vi "BRig_RT__Case_Exp__State_initTrial__LC_Select__v18.vi"(6 "input_arrTrig":bool[](array[boolean]), 8 "input_dataTrial":u16[][](array[numeric]), 9 "input_dataExp":u16[](array[numeric]), 10 "input_dataLC":u16[](array[numeric]), 11 "input_dataCurrent":u16[](array[numeric])) -> (0 "output_dataTrial":u16[][](array[numeric]), 3 "output_dataCurrent":u16[](array[numeric]), 4 "output_arrTrig":bool[](array[boolean]))   [LabVIEW 2014]
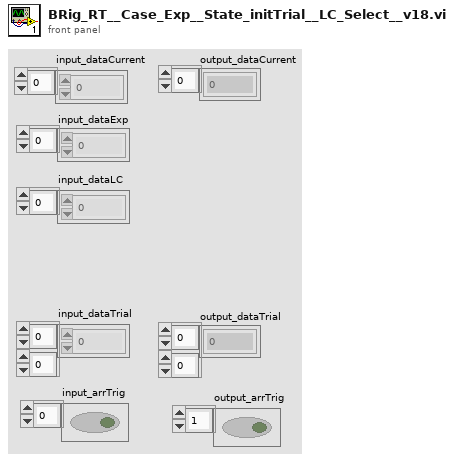
[diagram p1: front panel]
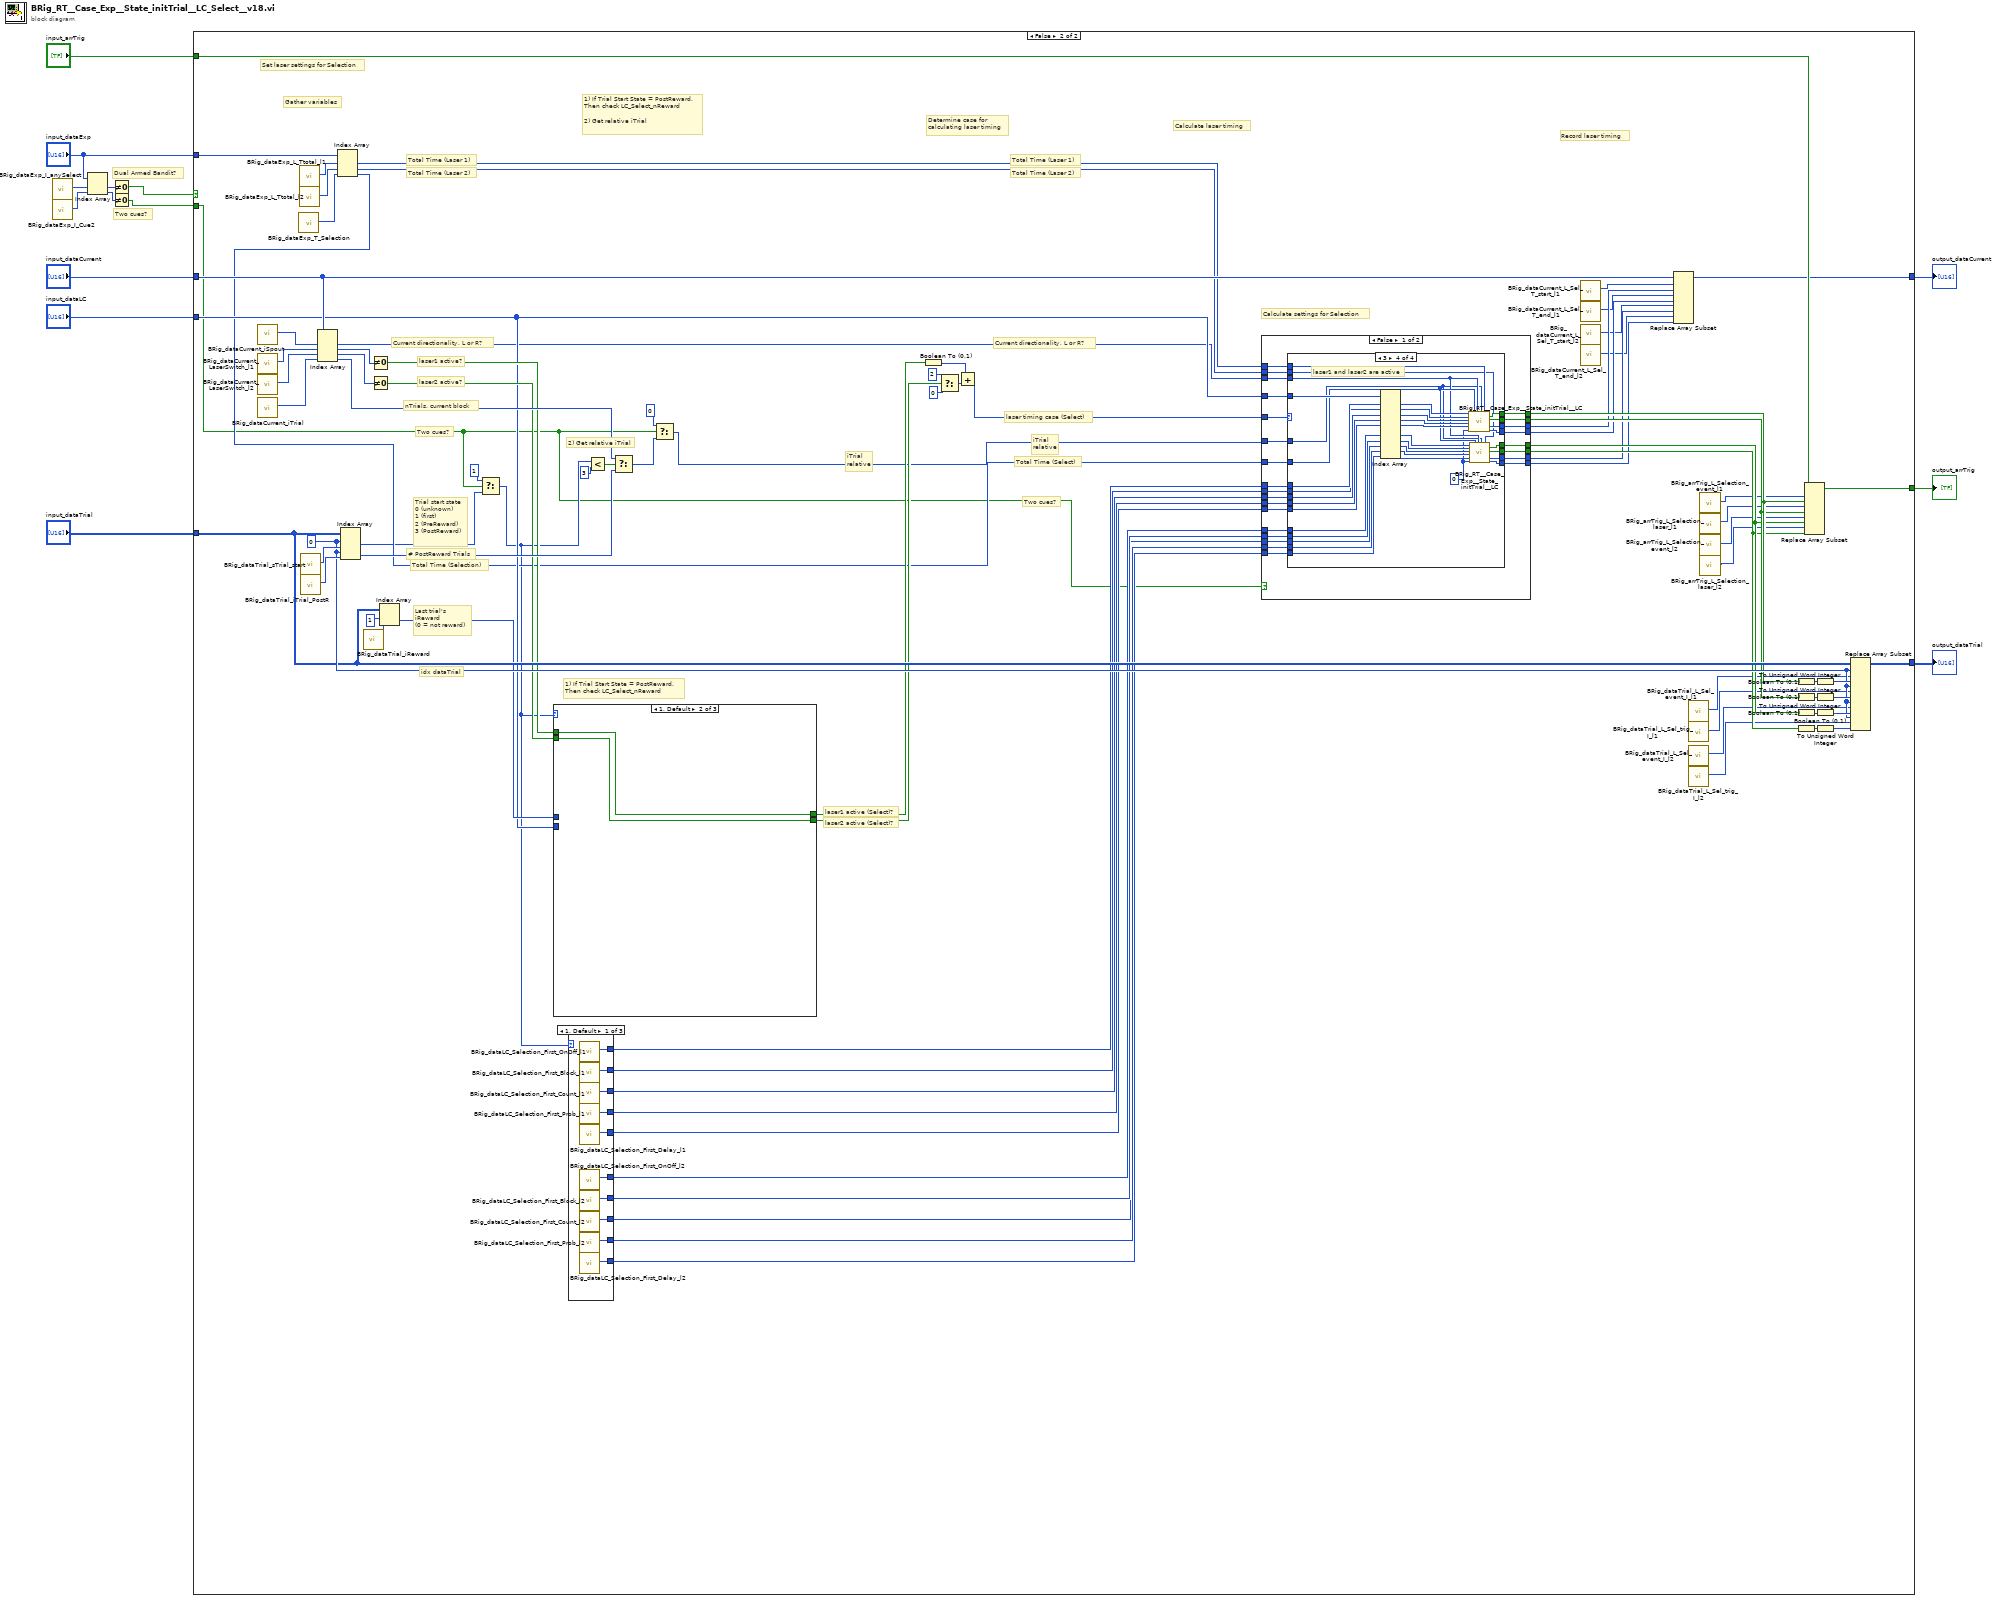
[diagram p0: block diagram]
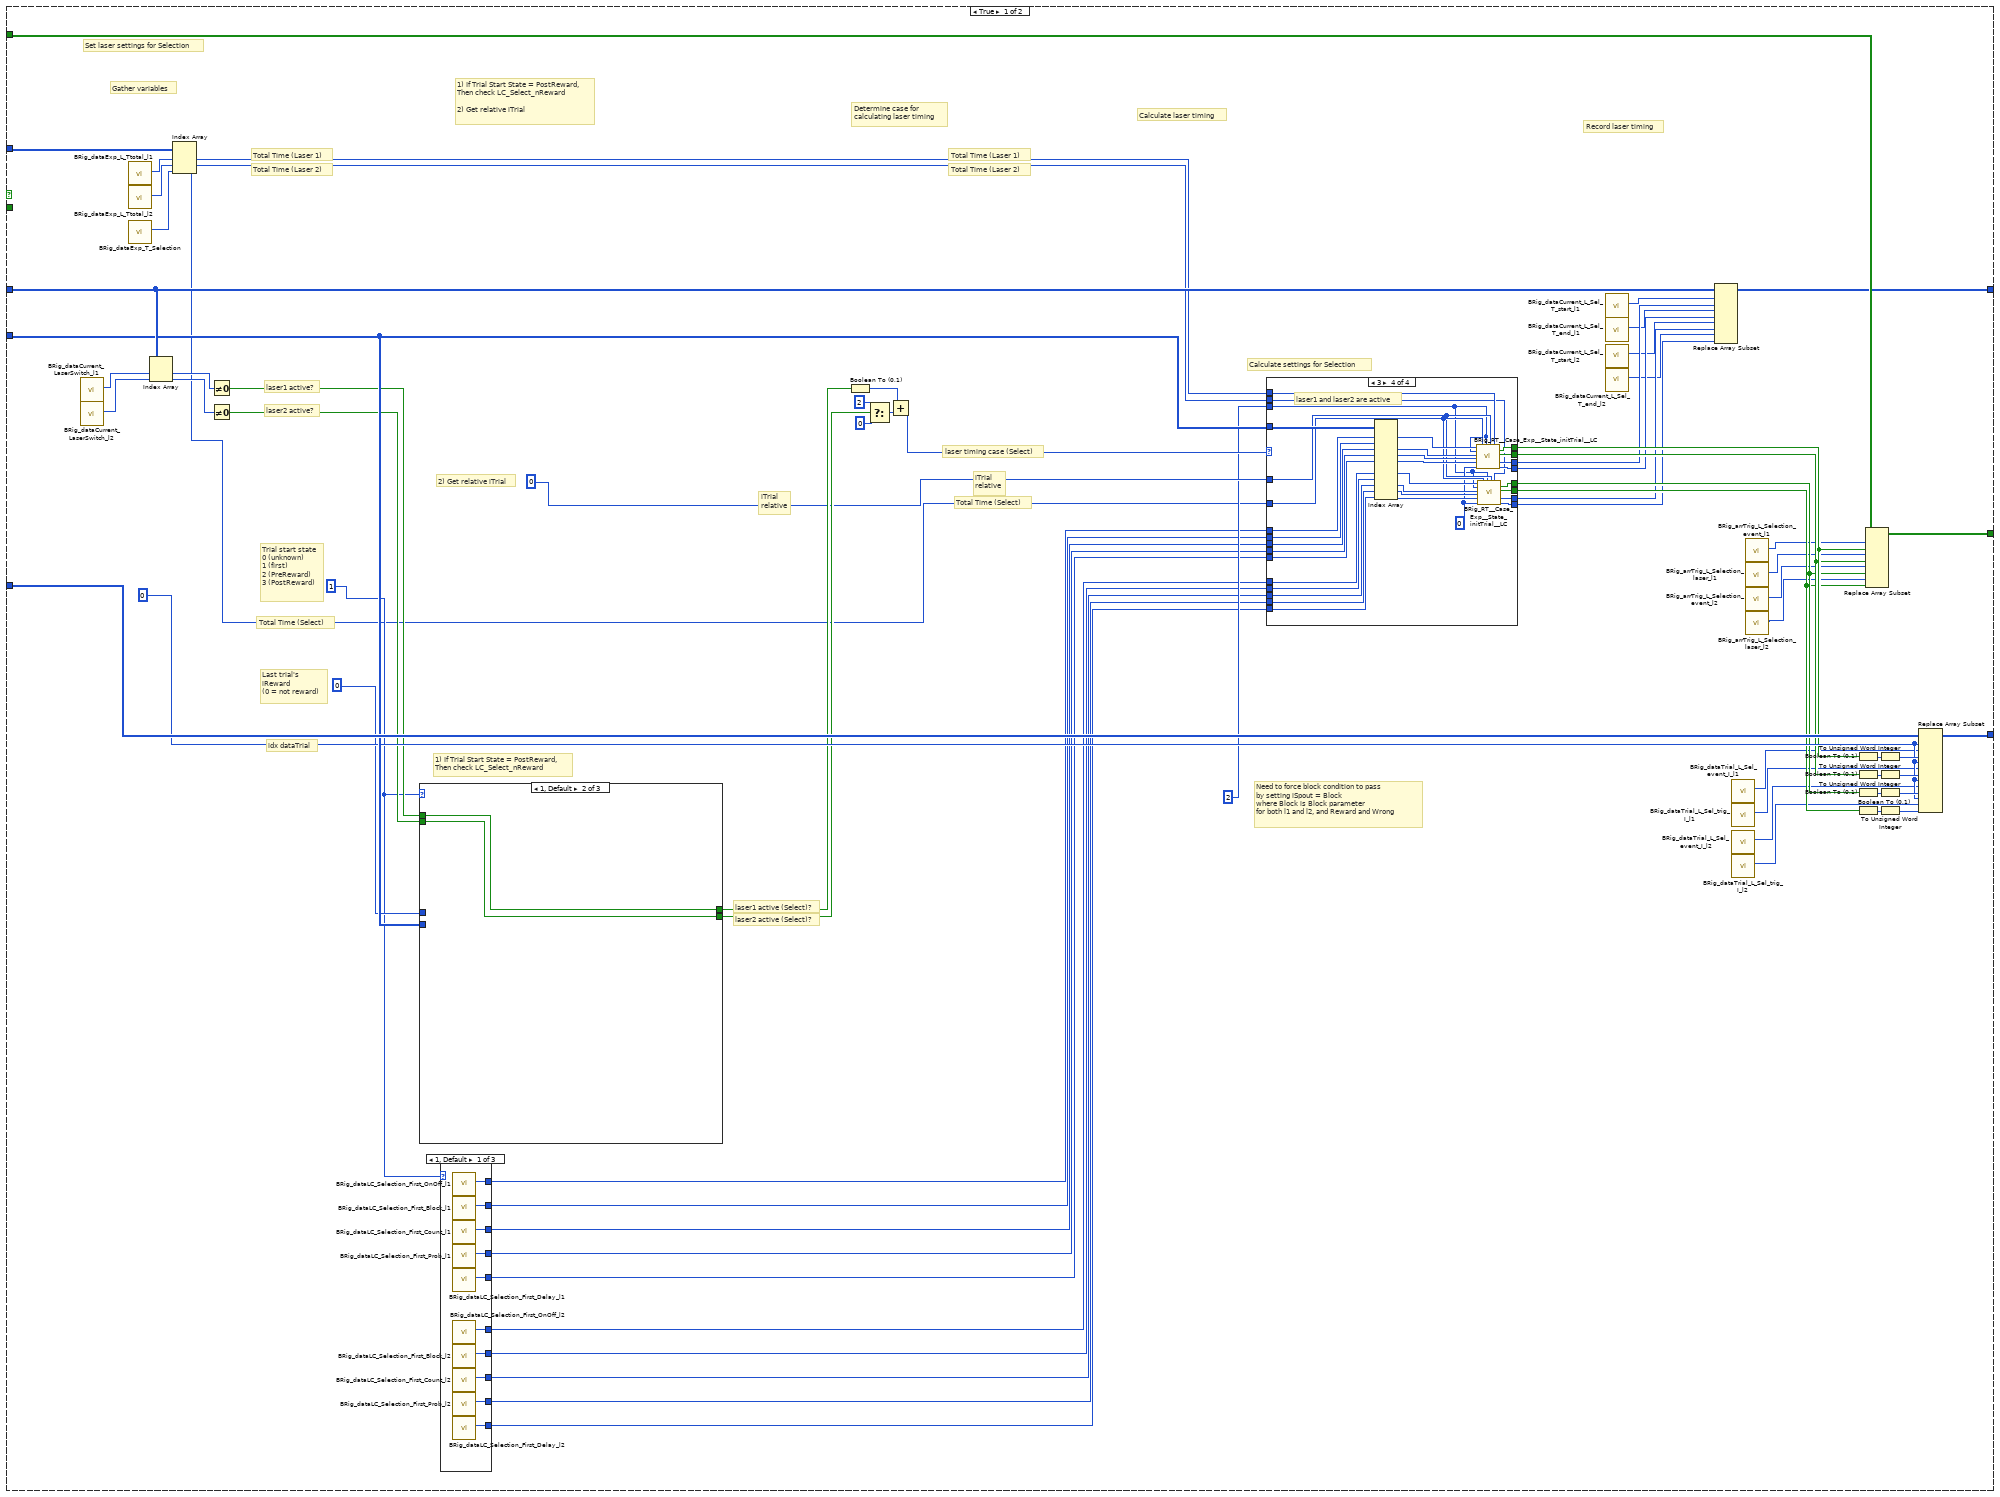
[diagram p2: hidden frame]
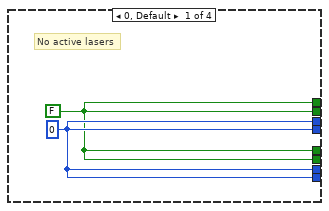
[diagram p3: hidden frame]
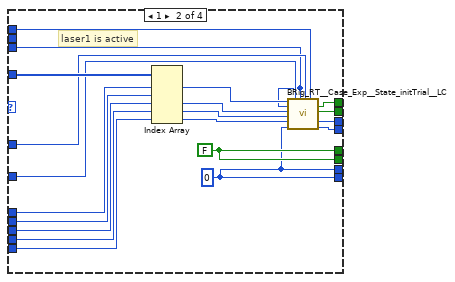
[diagram p4: hidden frame]
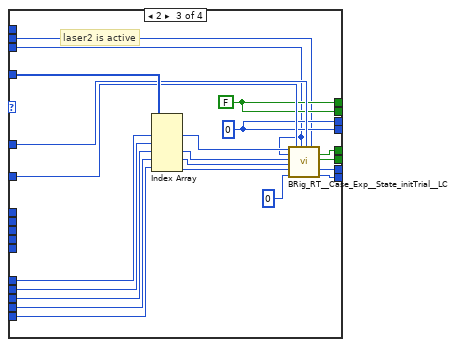
[diagram p5: hidden frame]
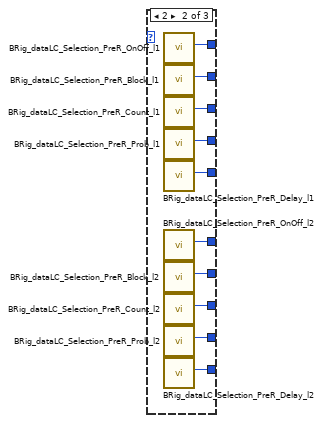
[diagram p6: hidden frame]
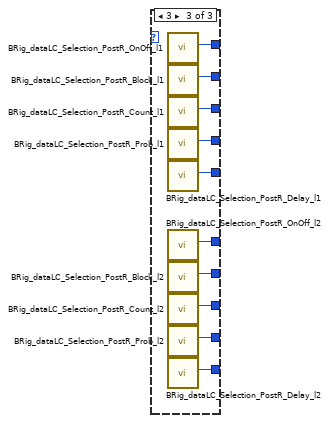
[diagram p7: hidden frame]
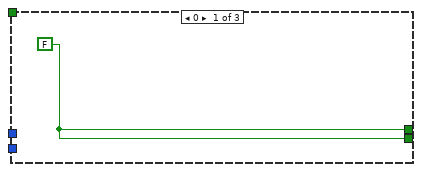
[diagram p8: hidden frame]
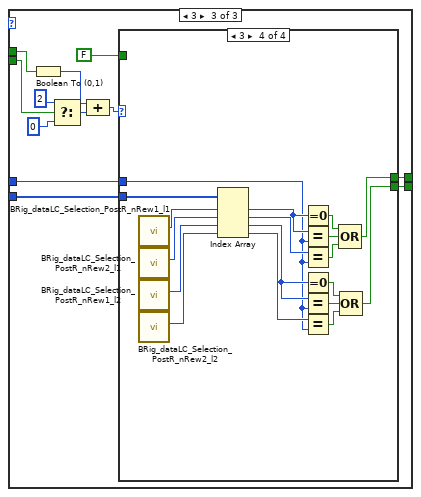
[diagram p9: hidden frame]
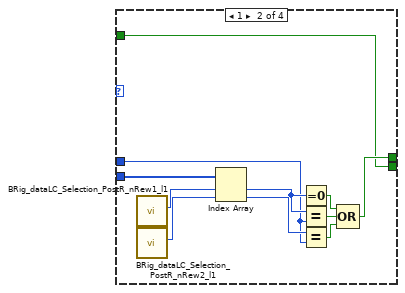
[diagram p11: hidden frame]
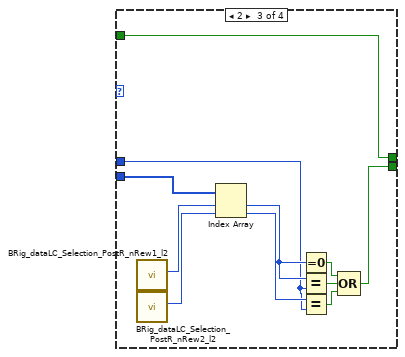
[diagram p12: hidden frame]
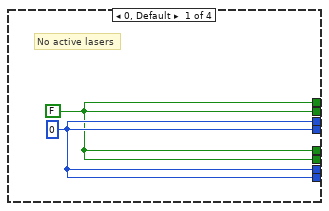
[diagram p13: hidden frame]
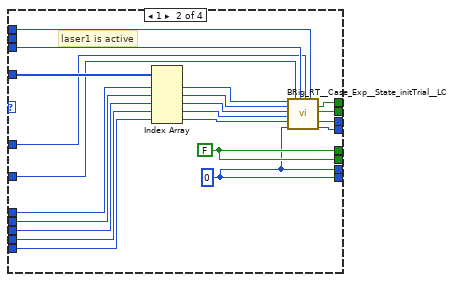
[diagram p14: hidden frame]
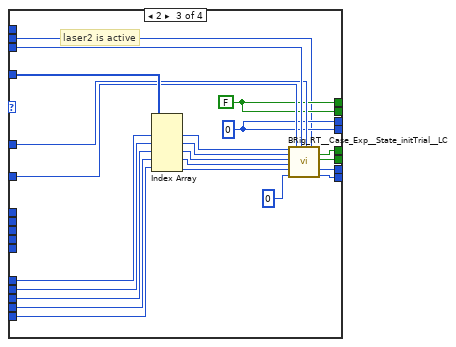
[diagram p15: hidden frame]
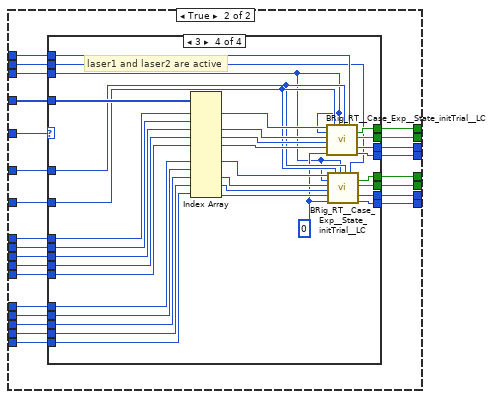
[diagram p16: hidden frame]
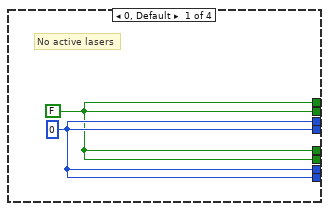
[diagram p17: hidden frame]
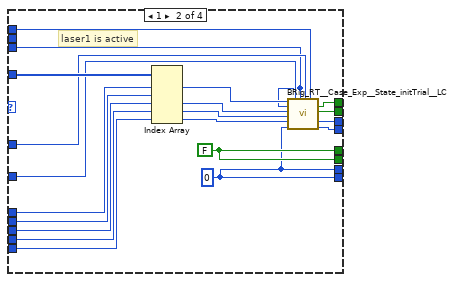
[diagram p18: hidden frame]
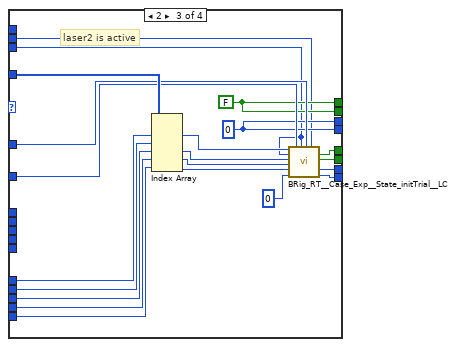
[diagram p19: hidden frame]
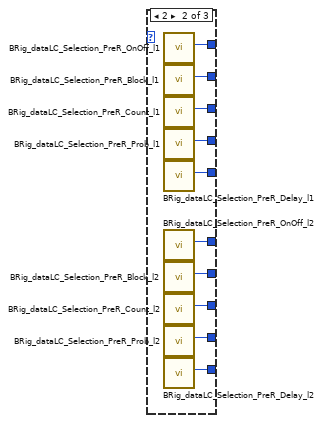
[diagram p20: hidden frame]
diagram:
  # "Two cues?"
  # "Dual Armed Bandit?"
  n1 = call "BRig_dataExp_I_anySelect.vi"() -> ("output_I_anySelect"=w7:i32)  [unwired: 11 in]
  n2 = call "BRig_dataExp_I_Cue2.vi"() -> ("output_I_Cue2"=w5:i32)  [unwired: 11 in]
  n3 = Index Array(array="input_dataExp", index #1=w7, index #2=w5) -> (element #1=w6:u16, element #2=w4:u16)
  n4 = Not Equal To 0?(x=w6) -> (x != 0?=w1:bool)
  n5 = Not Equal To 0?(x=w4) -> (x != 0?=w2:bool)
  n6 = case shown="False" w1 {
    tunnel: "input_arrTrig" -> [w84 w321]
    tunnel: [w83 w320] -> w13
    tunnel: [w82 w311] -> w12
    tunnel: "input_dataCurrent" -> [w81 w310]
    tunnel: [w80 w309] -> w10
    tunnel: "input_dataExp" -> [w79 w306]
    tunnel: "input_dataTrial" -> [w78 w300]
    tunnel: "input_dataLC" -> [w77 w288]
    tunnel: w2 -> [_ w247]
    frame True {
      w51 = u16 1
      w58 = 0
      # "Need to force block condition to pass\nby setting iSpout = Block\nwhere Block is Block parameter\nfor both l1 and l2, and Reward and Wrong"
      # "Record laser timing"
      # "Calculate laser timing"
      # "Total Time (Select)"
      # "iTrial\nrelative"
      # "Total Time (Laser 2)"
      # "Total Time (Laser 1)"
      # "Determine case for\ncalculating laser timing"
      # "2) Get relative iTrial"
      # "1) If Trial Start State = PostReward,\nThen check LC_Select_nReward"
      # "laser2 active (Select)?"
      # "laser1 active (Select)?"
      # "1) If Trial Start State = PostReward,\nThen check LC_Select_nReward\n\n2) Get relative iTrial"
      # "Gather variables"
      # "Last trial's\niReward\n(0 = not reward)"
      # "idx dataTrial"
      # "Total Time (Select)"
      # "Total Time (Laser 2)"
      # "Total Time (Laser 1)"
      # "Calculate settings for Selection"
      # "Set laser settings for Selection"
      # "iTrial\nrelative"
      # "laser timing case (Select)"
      # "Trial start state\n0 (unknown)\n1 (first)\n2 (PreReward)\n3 (PostReward)"
      # "laser2 active?"
      # "laser1 active?"
      n7 = call "BRig_dataCurrent_LaserSwitch_l1.vi"() -> ("output_LaserSwitch_l1"=w76:i32)  [unwired: 11 in]
      n8 = call "BRig_dataCurrent_LaserSwitch_l2.vi"() -> ("output_LaserSwitch_l2"=w75:i32)  [unwired: 11 in]
      n9 = call "BRig_dataExp_L_Ttotal_l1.vi"() -> ("output_L_Ttotal_l1"=w59:i32)  [unwired: 11 in]
      n10 = call "BRig_dataExp_L_Ttotal_l2.vi"() -> ("output_L_Ttotal_l2"=w60:i32)  [unwired: 11 in]
      n11 = call "BRig_dataExp_T_Selection.vi"() -> ("output_T_Selection"=w57:i32)  [unwired: 11 in]
      n12 = Index Array(array=w81, index #1=w76, index #2=w75) -> (element #1=w74:u16, element #2=w73:u16)
      n13 = Index Array(array=w79, index #1=w59, index #2=w60, index #3=w57) -> (element #1=w46:u16, element #2=w47:u16, element #3=w45:u16)
      n14 = Not Equal To 0?(x=w74) -> (x != 0?=w56:bool)
      n15 = Not Equal To 0?(x=w73) -> (x != 0?=w55:bool)
      n16 = case shown="1, Default" w51 {
        tunnel: u16 0 -> [_ _ w199]
        tunnel: w77 -> [_ _ w200]
        tunnel: w55 -> [_ w192 w194]
        tunnel: w56 -> [_ w193 w195]
        tunnel: [w191 w193 w198] -> w53
        tunnel: [w191 w192 w197] -> w52
        frame 0 {
          w191 = FALSE
        }
        frame 1, Default {
        }
        frame 3 {
          n17 = Boolean To (0,1)(Boolean=w195) -> (0, 1=w202:i16)
          n18 = Select(t=i16 2, s=w194, f=i16 0) -> (s? t:f=w203:i16)
          n19 = Compound Arithmetic op=ADD(w202, w203) -> (w201:i16)
          n20 = case shown="3" w201 {
            tunnel: w200 -> [_ w212 w223 w236]
            tunnel: w199 -> [_ w211 w222 w235]
            tunnel: [w206 w210 w220 w234] -> w198
            tunnel: [w206 w209 w221 w233] -> w197
            tunnel: FALSE -> [w206 w209 w220 _]
            frame 0, Default {
            }
            frame 1 {
              n21 = call "BRig_dataLC_Selection_PostR_nRew1_l1.vi"() -> ("output_Selection_PostR_nRew1_l1"=w207:i32)  [unwired: 11 in]
              n22 = call "BRig_dataLC_Selection_PostR_nRew2_l1.vi"() -> ("output_Selection_PostR_nRew2_l1"=w208:i32)  [unwired: 11 in]
              n23 = Index Array(array=w212, index #1=w207, index #2=w208) -> (element #1=w214:u16, element #2=w213:u16)
              n24 = Equal To 0?(x=w214) -> (x = 0?=w215:bool)
              n25 = Equal?(x=w214, y=w211) -> (x = y?=w216:bool)
              n26 = Equal?(x=w213, y=w211) -> (x = y?=w217:bool)
              n27 = Compound Arithmetic op=OR(w215, w216, w217) -> (w210:bool)
            }
            frame 2 {
              n28 = call "BRig_dataLC_Selection_PostR_nRew1_l2.vi"() -> ("output_Selection_PostR_nRew1_l2"=w218:i32)  [unwired: 11 in]
              n29 = call "BRig_dataLC_Selection_PostR_nRew2_l2.vi"() -> ("output_Selection_PostR_nRew2_l2"=w219:i32)  [unwired: 11 in]
              n30 = Index Array(array=w223, index #1=w218, index #2=w219) -> (element #1=w224:u16, element #2=w225:u16)
              n31 = Equal To 0?(x=w224) -> (x = 0?=w227:bool)
              n32 = Equal?(x=w224, y=w222) -> (x = y?=w226:bool)
              n33 = Equal?(x=w225, y=w222) -> (x = y?=w228:bool)
              n34 = Compound Arithmetic op=OR(w227, w226, w228) -> (w221:bool)
            }
            frame 3 {
              n35 = call "BRig_dataLC_Selection_PostR_nRew1_l1.vi"() -> ("output_Selection_PostR_nRew1_l1"=w229:i32)  [unwired: 11 in]
              n36 = call "BRig_dataLC_Selection_PostR_nRew2_l1.vi"() -> ("output_Selection_PostR_nRew2_l1"=w230:i32)  [unwired: 11 in]
              n37 = call "BRig_dataLC_Selection_PostR_nRew1_l2.vi"() -> ("output_Selection_PostR_nRew1_l2"=w231:i32)  [unwired: 11 in]
              n38 = call "BRig_dataLC_Selection_PostR_nRew2_l2.vi"() -> ("output_Selection_PostR_nRew2_l2"=w232:i32)  [unwired: 11 in]
              n39 = Index Array(array=w236, index #1=w229, index #2=w230, index #3=w231, index #4=w232) -> (element #1=w240:u16, element #2=w239:u16, element #3=w237:u16, element #4=w238:u16)
              n40 = Equal To 0?(x=w240) -> (x = 0?=w241:bool)
              n41 = Equal?(x=w240, y=w235) -> (x = y?=w242:bool)
              n42 = Equal?(x=w239, y=w235) -> (x = y?=w243:bool)
              n43 = Equal To 0?(x=w237) -> (x = 0?=w245:bool)
              n44 = Equal?(x=w237, y=w235) -> (x = y?=w244:bool)
              n45 = Equal?(x=w238, y=w235) -> (x = y?=w246:bool)
              n46 = Compound Arithmetic op=OR(w241, w242, w243) -> (w234:bool)
              n47 = Compound Arithmetic op=OR(w245, w244, w246) -> (w233:bool)
            }
          }
        }
      }
      n48 = case shown="1, Default" w51 {
        tunnel: [w170 w180 w190] -> w44
        tunnel: [w163 w178 w188] -> w43
        tunnel: [w164 w177 w187] -> w42
        tunnel: [w165 w176 w186] -> w41
        tunnel: [w166 w175 w185] -> w40
        tunnel: [w169 w179 w189] -> w39
        tunnel: [w167 w174 w184] -> w38
        tunnel: [w168 w173 w183] -> w37
        tunnel: [w161 w172 w182] -> w36
        tunnel: [w162 w171 w181] -> w35
        frame 1, Default {
          n49 = call "BRig_dataLC_Selection_First_OnOff_l1.vi"() -> ("output_Selection_First_OnOff"=w170:i32)  [unwired: 11 in]
          n50 = call "BRig_dataLC_Selection_First_Block_l1.vi"() -> ("output_Selection_First_Block"=w163:i32)  [unwired: 11 in]
          n51 = call "BRig_dataLC_Selection_First_Count_l1.vi"() -> ("output_Selection_First_Count"=w164:i32)  [unwired: 11 in]
          n52 = call "BRig_dataLC_Selection_First_Prob_l1.vi"() -> ("output_Selection_First_Prob"=w165:i32)  [unwired: 11 in]
          n53 = call "BRig_dataLC_Selection_First_Delay_l1.vi"() -> ("output_Selection_First_Delay"=w166:i32)  [unwired: 11 in]
          n54 = call "BRig_dataLC_Selection_First_OnOff_l2.vi"() -> ("output_Selection_First_OnOff_l2"=w169:i32)  [unwired: 11 in]
          n55 = call "BRig_dataLC_Selection_First_Block_l2.vi"() -> ("output_Selection_First_Block_l2"=w167:i32)  [unwired: 11 in]
          n56 = call "BRig_dataLC_Selection_First_Count_l2.vi"() -> ("output_Selection_First_Count_l2"=w168:i32)  [unwired: 11 in]
          n57 = call "BRig_dataLC_Selection_First_Prob_l2.vi"() -> ("output_Selection_First_Prob_l2"=w161:i32)  [unwired: 11 in]
          n58 = call "BRig_dataLC_Selection_First_Delay_l2.vi"() -> ("output_Selection_First_Delay_l2"=w162:i32)  [unwired: 11 in]
        }
        frame 2 {
          n59 = call "BRig_dataLC_Selection_PreR_OnOff_l1.vi"() -> ("output_Selection_PreR_OnOff"=w180:i32)  [unwired: 11 in]
          n60 = call "BRig_dataLC_Selection_PreR_Block_l1.vi"() -> ("output_Selection_PreR_Block"=w178:i32)  [unwired: 11 in]
          n61 = call "BRig_dataLC_Selection_PreR_Count_l1.vi"() -> ("output_Selection_PreR_Count"=w177:i32)  [unwired: 11 in]
          n62 = call "BRig_dataLC_Selection_PreR_Prob_l1.vi"() -> ("output_Selection_PreR_Prob"=w176:i32)  [unwired: 11 in]
          n63 = call "BRig_dataLC_Selection_PreR_Delay_l1.vi"() -> ("output_Selection_PreR_Delay"=w175:i32)  [unwired: 11 in]
          n64 = call "BRig_dataLC_Selection_PreR_OnOff_l2.vi"() -> ("output_Selection_PreR_OnOff_l2"=w179:i32)  [unwired: 11 in]
          n65 = call "BRig_dataLC_Selection_PreR_Block_l2.vi"() -> ("output_Selection_PreR_Block_l2"=w174:i32)  [unwired: 11 in]
          n66 = call "BRig_dataLC_Selection_PreR_Count_l2.vi"() -> ("output_Selection_PreR_Count_l2"=w173:i32)  [unwired: 11 in]
          n67 = call "BRig_dataLC_Selection_PreR_Prob_l2.vi"() -> ("output_Selection_PreR_Prob_l2"=w172:i32)  [unwired: 11 in]
          n68 = call "BRig_dataLC_Selection_PreR_Delay_l2.vi"() -> ("output_Selection_PreR_Delay_l2"=w171:i32)  [unwired: 11 in]
        }
        frame 3 {
          n69 = call "BRig_dataLC_Selection_PostR_OnOff_l1.vi"() -> ("output_Selection_PostR_OnOff"=w190:i32)  [unwired: 11 in]
          n70 = call "BRig_dataLC_Selection_PostR_Block_l1.vi"() -> ("output_Selection_PostR_Block"=w188:i32)  [unwired: 11 in]
          n71 = call "BRig_dataLC_Selection_PostR_Count_l1.vi"() -> ("output_Selection_PostR_Count"=w187:i32)  [unwired: 11 in]
          n72 = call "BRig_dataLC_Selection_PostR_Prob_l1.vi"() -> ("output_Selection_PostR_Prob"=w186:i32)  [unwired: 11 in]
          n73 = call "BRig_dataLC_Selection_PostR_Delay_l1.vi"() -> ("output_Selection_PostR_Delay"=w185:i32)  [unwired: 11 in]
          n74 = call "BRig_dataLC_Selection_PostR_OnOff_l2.vi"() -> ("output_Selection_PostR_OnOff_l2"=w189:i32)  [unwired: 11 in]
          n75 = call "BRig_dataLC_Selection_PostR_Block_l2.vi"() -> ("output_Selection_PostR_Block_l2"=w184:i32)  [unwired: 11 in]
          n76 = call "BRig_dataLC_Selection_PostR_Count_l2.vi"() -> ("output_Selection_PostR_Count_l2"=w183:i32)  [unwired: 11 in]
          n77 = call "BRig_dataLC_Selection_PostR_Prob_l2.vi"() -> ("output_Selection_PostR_Prob_l2"=w182:i32)  [unwired: 11 in]
          n78 = call "BRig_dataLC_Selection_PostR_Delay_l2.vi"() -> ("output_Selection_PostR_Delay_l2"=w181:i32)  [unwired: 11 in]
        }
      }
      n79 = Boolean To (0,1)(Boolean=w53) -> (0, 1=w70:i16)
      n80 = Select(t=i16 2, s=w52, f=i16 0) -> (s? t:f=w71:i16)
      n81 = Add(x=w70, y=w71) -> (x+y=w50:i16)
      n82 = case shown="3" w50 {
        tunnel: w77 -> [_ w106 w127 w160]
        tunnel: u16 2 ("input_sState_start") -> [_ w87 w107 w128]
        tunnel: w45 -> [_ w101 w122 w151]
        tunnel: u16 0 -> [_ w100 w121 w150]
        tunnel: [w85 w99 w111 w149] -> w34
        tunnel: [w85 w98 w111 w148] -> w33
        tunnel: [w86 w97 w110 w147] -> w32
        tunnel: [w86 w96 w110 w146] -> w31
        tunnel: [w85 w90 w120 w145] -> w29
        tunnel: [w86 w88 w119 w144] -> w28
        tunnel: [w85 w90 w118 w143] -> w30
        tunnel: [w86 w88 w117 w142] -> w27
        tunnel: w44 -> [_ w95 _ w141]
        tunnel: w43 -> [_ w94 _ w140]
        tunnel: w42 -> [_ w93 _ w139]
        tunnel: w41 -> [_ w92 _ w138]
        tunnel: w40 -> [_ w91 _ w137]
        tunnel: w39 -> [_ _ w116 w136]
        tunnel: w38 -> [_ _ w115 w135]
        tunnel: w37 -> [_ _ w114 w134]
        tunnel: w36 -> [_ _ w113 w133]
        tunnel: w35 -> [_ _ w112 w132]
        tunnel: w46 -> [_ w89 _ w131]
        tunnel: w47 -> [_ _ w109 w130]
        frame 0, Default {
          w86 = u16 0
          w85 = FALSE
          # "No active lasers"
        }
        frame 1 {
          w88 = u16 0
          w90 = FALSE
          # "laser1 is active"
          n83 = Index Array(array=w106, index #1=w95, index #2=w94, index #3=w93, index #4=w92, index #5=w91) -> (element #1=w105:u16, element #3=w104:u16, element #4=w103:u16, element #5=w102:u16)  [unwired: 1 out]
          n84 = call "BRig_RT__Case_Exp__State_initTrial__LC.vi"("input_L_OnOff"=w105, "input_L_Block"=w87, "input_L_Count"=w104, "input_L_Prob"=w103, "input_L_Tdelay"=w102, "input_L_delayOpt"=w88, "input_T_state"=w101, "input_iSpout"=w87, "input_iTrial_relative"=w100, "input_L_T"=w89) -> ("output_LC_Event"=w99:bool, "output_LC_Laser"=w98:bool, "output_L_Tstart"=w97:u16, "output_L_Tend"=w96:u16)  [unwired: 6 in]
        }
        frame 2 {
          w110 = u16 0
          w111 = FALSE
          # "laser2 is active"
          n85 = Index Array(array=w127, index #1=w116, index #2=w115, index #3=w114, index #4=w113, index #5=w112) -> (element #1=w123:u16, element #3=w124:u16, element #4=w125:u16, element #5=w126:u16)  [unwired: 1 out]
          n86 = call "BRig_RT__Case_Exp__State_initTrial__LC.vi"("input_L_OnOff"=w123, "input_L_Block"=w107, "input_L_Count"=w124, "input_L_Prob"=w125, "input_L_Tdelay"=w126, "input_L_delayOpt"=u16 0, "input_T_state"=w122, "input_iSpout"=w107, "input_iTrial_relative"=w121, "input_L_T"=w109) -> ("output_LC_Event"=w118:bool, "output_LC_Laser"=w120:bool, "output_L_Tstart"=w119:u16, "output_L_Tend"=w117:u16)  [unwired: 6 in]
        }
        frame 3 {
          w129 = u16 0 ("input_L_delayOpt")
          # "laser1 and laser2 are active"
          n87 = Index Array(array=w160, index #1=w141, index #2=w140, index #3=w139, index #4=w138, index #5=w137, index #7=w136, index #8=w135, index #9=w134, index #10=w133, index #11=w132) -> (element #1=w159:u16, element #3=w158:u16, element #4=w157:u16, element #5=w156:u16, element #7=w152:u16, element #9=w153:u16, element #10=w154:u16, element #11=w155:u16)  [unwired: 1 in, 3 out]
          n88 = call "BRig_RT__Case_Exp__State_initTrial__LC.vi"("input_L_OnOff"=w159, "input_L_Block"=w128, "input_L_Count"=w158, "input_L_Prob"=w157, "input_L_Tdelay"=w156, "input_L_delayOpt"=w129, "input_T_state"=w151, "input_iSpout"=w128, "input_iTrial_relative"=w150, "input_L_T"=w131) -> ("output_LC_Event"=w149:bool, "output_LC_Laser"=w148:bool, "output_L_Tstart"=w147:u16, "output_L_Tend"=w146:u16)  [unwired: 6 in]
          n89 = call "BRig_RT__Case_Exp__State_initTrial__LC.vi"("input_L_OnOff"=w152, "input_L_Block"=w128, "input_L_Count"=w153, "input_L_Prob"=w154, "input_L_Tdelay"=w155, "input_L_delayOpt"=w129, "input_T_state"=w151, "input_iSpout"=w128, "input_iTrial_relative"=w150, "input_L_T"=w130) -> ("output_LC_Event"=w143:bool, "output_LC_Laser"=w145:bool, "output_L_Tstart"=w144:u16, "output_L_Tend"=w142:u16)  [unwired: 6 in]
        }
      }
      n90 = call "BRig_dataCurrent_L_Sel_T_start_l1.vi"() -> ("output_L_Sel_T_start_l1"=w26:i32)  [unwired: 11 in]
      n91 = call "BRig_dataCurrent_L_Sel_T_end_l1.vi"() -> ("output_L_Sel_T_end_l1"=w25:i32)  [unwired: 11 in]
      n92 = call "BRig_dataCurrent_L_Sel_T_start_l2.vi"() -> ("output_L_Sel_T_start_l2"=w24:i32)  [unwired: 11 in]
      n93 = call "BRig_dataCurrent_L_Sel_T_end_l2.vi"() -> ("output_L_Sel_T_end_l2"=w23:i32)  [unwired: 11 in]
      n94 = Replace Array Subset(array=w81, new element #1=w32, index #1=w26, new element #2=w31, index #2=w25, new element #3=w28, index #3=w24, new element #4=w27, index #4=w23) -> (w80:u16[])
      n95 = call "BRig_dataTrial_L_Sel_event_I_l1.vi"() -> ("output_L_Sel_event_I_l1"=w18:i32)  [unwired: 11 in]
      n96 = call "BRig_dataTrial_L_Sel_trig_I_l1.vi"() -> ("output_L_Sel_trig_I_l1"=w17:i32)  [unwired: 11 in]
      n97 = call "BRig_dataTrial_L_Sel_event_I_l2.vi"() -> ("output_L_Sel_event_I_l2"=w16:i32)  [unwired: 11 in]
      n98 = call "BRig_dataTrial_L_Sel_trig_I_l2.vi"() -> ("output_L_Sel_trig_I_l2"=w15:i32)  [unwired: 11 in]
      n99 = call "BRig_arrTrig_L_Selection_event_l1.vi"() -> ("output_L_Sel_event_l1"=w22:i32)  [unwired: 11 in]
      n100 = call "BRig_arrTrig_L_Selection_laser_l1.vi"() -> ("output_L_Sel_laserTrig_l1"=w21:i32)  [unwired: 11 in]
      n101 = call "BRig_arrTrig_L_Selection_event_l2.vi"() -> ("output_L_Sel_event_l2"=w20:i32)  [unwired: 11 in]
      n102 = call "BRig_arrTrig_L_Selection_laser_l2.vi"() -> ("output_L_Sel_laserTrig_l2"=w19:i32)  [unwired: 11 in]
      n103 = Boolean To (0,1)(Boolean=w34) -> (0, 1=w68:i16)
      n104 = Boolean To (0,1)(Boolean=w33) -> (0, 1=w67:i16)
      n105 = Boolean To (0,1)(Boolean=w30) -> (0, 1=w65:i16)
      n106 = Boolean To (0,1)(Boolean=w29) -> (0, 1=w66:i16)
      n107 = Replace Array Subset(array=w84, new element #1=w34, index #1=w22, new element #2=w33, index #2=w21, new element #3=w30, index #3=w20, new element #4=w29, index #4=w19) -> (w83:bool[])
      n108 = To Unsigned Word Integer(number=w68) -> (unsigned 16bit integer=w64:u16)
      n109 = To Unsigned Word Integer(number=w67) -> (unsigned 16bit integer=w63:u16)
      n110 = To Unsigned Word Integer(number=w65) -> (unsigned 16bit integer=w62:u16)
      n111 = To Unsigned Word Integer(number=w66) -> (unsigned 16bit integer=w61:u16)
      n112 = Replace Array Subset(array=w78, new element #1=w64, index (row) #1=w58, index (col) #1=w18, new element #2=w63, index (row) #2=w58, index (col) #2=w17, new element #3=w62, index (row) #3=w58, index (col) #3=w16, new element #4=w61, index (row) #4=w58, index (col) #4=w15) -> (w82:u16[][])
    }
    frame False {
      w303 = 0
      # "Two cues?"
      # "Two cues?"
      # "Record laser timing"
      # "Calculate laser timing"
      # "Total Time (Select)"
      # "iTrial\nrelative"
      # "Total Time (Laser 2)"
      # "Total Time (Laser 1)"
      # "Current directionality, L or R?"
      # "Determine case for\ncalculating laser timing"
      # "2) Get relative iTrial"
      # "1) If Trial Start State = PostReward,\nThen check LC_Select_nReward"
      # "laser2 active (Select)?"
      # "laser1 active (Select)?"
      # "1) If Trial Start State = PostReward,\nThen check LC_Select_nReward\n\n2) Get relative iTrial"
      # "Gather variables"
      # "Last trial's\niReward\n(0 = not reward)"
      # "nTrials, current block"
      # "idx dataTrial"
      # "Total Time (Selection)"
      # "# PostReward Trials"
      # "Current directionality, L or R?"
      # "Total Time (Laser 2)"
      # "Total Time (Laser 1)"
      # "Calculate settings for Selection"
      # "Set laser settings for Selection"
      # "iTrial\nrelative"
      # "laser timing case (Select)"
      # "Trial start state\n0 (unknown)\n1 (first)\n2 (PreReward)\n3 (PostReward)"
      # "laser2 active?"
      # "laser1 active?"
      n113 = call "BRig_dataCurrent_iSpout.vi"() -> ("output_iSpout"=w322:i32)  [unwired: 11 in]
      n114 = call "BRig_dataCurrent_LaserSwitch_l1.vi"() -> ("output_LaserSwitch_l1"=w331:i32)  [unwired: 11 in]
      n115 = call "BRig_dataCurrent_LaserSwitch_l2.vi"() -> ("output_LaserSwitch_l2"=w330:i32)  [unwired: 11 in]
      n116 = call "BRig_dataCurrent_iTrial.vi"() -> ("output_iTrial"=w304:i32)  [unwired: 11 in]
      n117 = call "BRig_dataExp_T_Selection.vi"() -> ("output_T_Selection"=w290:i32)  [unwired: 11 in]
      n118 = call "BRig_dataExp_L_Ttotal_l1.vi"() -> ("output_L_Ttotal_l1"=w307:i32)  [unwired: 11 in]
      n119 = call "BRig_dataExp_L_Ttotal_l2.vi"() -> ("output_L_Ttotal_l2"=w308:i32)  [unwired: 11 in]
      n120 = call "BRig_dataTrial_sTrial_start.vi"() -> ("output_sTrial_start"=w327:i32)  [unwired: 11 in]
      n121 = call "BRig_dataTrial_iTrial_PostR.vi"() -> ("output_iTrial_PostR"=w305:i32)  [unwired: 11 in]
      n122 = Index Array(array=w310, index #1=w322, index #2=w331, index #3=w330, index #4=w304) -> (element #1=w276:u16, element #2=w329:u16, element #3=w328:u16, element #4=w297:u16)
      n123 = Index Array(array=w306, index #1=w307, index #2=w308, index #3=w290) -> (element #1=w274:u16, element #2=w275:u16, element #3=w287:u16)
      n124 = Index Array(array=w300, index (row) #1=w303, index (col) #1=w327, index (row) #2=w303, index (col) #2=w305) -> (element #1=w252:u16, element #2=w296:u16)
      n125 = call "BRig_dataTrial_iReward.vi"() -> ("output_iReward"=w301:i32)  [unwired: 11 in]
      n126 = Not Equal To 0?(x=w329) -> (x != 0?=w295:bool)
      n127 = Not Equal To 0?(x=w328) -> (x != 0?=w294:bool)
      n128 = Index Array(array=w300, index (row)=1 ("disabled index (row)"), index (col)=w301) -> (element=w293:u16)
      n129 = Select(t=u16 1, s=w247, f=w252) -> (s? t:f=w251:u16)
      n130 = case shown="1, Default" w251 {
        tunnel: w293 -> [_ _ w576]
        tunnel: w288 -> [_ _ w575]
        tunnel: w294 -> [_ w569 w577]
        tunnel: w295 -> [_ w570 w578]
        tunnel: [w568 w570 w574] -> w292
        tunnel: [w568 w569 w571] -> w291
        frame 0 {
          w568 = FALSE
        }
        frame 1, Default {
        }
        frame 3 {
          n131 = Boolean To (0,1)(Boolean=w578) -> (0, 1=w579:i16)
          n132 = Select(t=i16 2, s=w577, f=i16 0) -> (s? t:f=w580:i16)
          n133 = Compound Arithmetic op=ADD(w579, w580) -> (w572:i16)
          n134 = case shown="1" w572 {
            tunnel: w575 -> [_ w589 w600 w613]
            tunnel: w576 -> [_ w588 w599 w612]
            tunnel: [w583 w587 w597 w611] -> w574
            tunnel: [w583 w586 w598 w610] -> w571
            tunnel: FALSE -> [w583 w586 w597 _]
            frame 0, Default {
            }
            frame 1 {
              n135 = call "BRig_dataLC_Selection_PostR_nRew1_l1.vi"() -> ("output_Selection_PostR_nRew1_l1"=w584:i32)  [unwired: 11 in]
              n136 = call "BRig_dataLC_Selection_PostR_nRew2_l1.vi"() -> ("output_Selection_PostR_nRew2_l1"=w585:i32)  [unwired: 11 in]
              n137 = Index Array(array=w589, index #1=w584, index #2=w585) -> (element #1=w591:u16, element #2=w590:u16)
              n138 = Equal To 0?(x=w591) -> (x = 0?=w592:bool)
              n139 = Equal?(x=w591, y=w588) -> (x = y?=w593:bool)
              n140 = Equal?(x=w590, y=w588) -> (x = y?=w594:bool)
              n141 = Compound Arithmetic op=OR(w592, w593, w594) -> (w587:bool)
            }
            frame 2 {
              n142 = call "BRig_dataLC_Selection_PostR_nRew1_l2.vi"() -> ("output_Selection_PostR_nRew1_l2"=w595:i32)  [unwired: 11 in]
              n143 = call "BRig_dataLC_Selection_PostR_nRew2_l2.vi"() -> ("output_Selection_PostR_nRew2_l2"=w596:i32)  [unwired: 11 in]
              n144 = Index Array(array=w600, index #1=w595, index #2=w596) -> (element #1=w601:u16, element #2=w602:u16)
              n145 = Equal To 0?(x=w601) -> (x = 0?=w604:bool)
              n146 = Equal?(x=w601, y=w599) -> (x = y?=w603:bool)
              n147 = Equal?(x=w602, y=w599) -> (x = y?=w605:bool)
              n148 = Compound Arithmetic op=OR(w604, w603, w605) -> (w598:bool)
            }
            frame 3 {
              n149 = call "BRig_dataLC_Selection_PostR_nRew1_l1.vi"() -> ("output_Selection_PostR_nRew1_l1"=w606:i32)  [unwired: 11 in]
              n150 = call "BRig_dataLC_Selection_PostR_nRew2_l1.vi"() -> ("output_Selection_PostR_nRew2_l1"=w607:i32)  [unwired: 11 in]
              n151 = call "BRig_dataLC_Selection_PostR_nRew1_l2.vi"() -> ("output_Selection_PostR_nRew1_l2"=w608:i32)  [unwired: 11 in]
              n152 = call "BRig_dataLC_Selection_PostR_nRew2_l2.vi"() -> ("output_Selection_PostR_nRew2_l2"=w609:i32)  [unwired: 11 in]
              n153 = Index Array(array=w613, index #1=w606, index #2=w607, index #3=w608, index #4=w609) -> (element #1=w617:u16, element #2=w616:u16, element #3=w614:u16, element #4=w615:u16)
              n154 = Equal To 0?(x=w617) -> (x = 0?=w618:bool)
              n155 = Equal?(x=w617, y=w612) -> (x = y?=w619:bool)
              n156 = Equal?(x=w616, y=w612) -> (x = y?=w620:bool)
              n157 = Equal To 0?(x=w614) -> (x = 0?=w622:bool)
              n158 = Equal?(x=w614, y=w612) -> (x = y?=w621:bool)
              n159 = Equal?(x=w615, y=w612) -> (x = y?=w623:bool)
              n160 = Compound Arithmetic op=OR(w618, w619, w620) -> (w611:bool)
              n161 = Compound Arithmetic op=OR(w622, w621, w623) -> (w610:bool)
            }
          }
        }
      }
      n162 = case shown="1, Default" w251 {
        tunnel: [w547 w557 w567] -> w286
        tunnel: [w540 w555 w558] -> w285
        tunnel: [w541 w554 w565] -> w284
        tunnel: [w542 w553 w564] -> w283
        tunnel: [w543 w552 w563] -> w282
        tunnel: [w546 w556 w566] -> w281
        tunnel: [w544 w551 w562] -> w280
        tunnel: [w545 w550 w561] -> w279
        tunnel: [w538 w549 w560] -> w278
        tunnel: [w539 w548 w559] -> w277
        frame 1, Default {
          n163 = call "BRig_dataLC_Selection_First_OnOff_l1.vi"() -> ("output_Selection_First_OnOff"=w547:i32)  [unwired: 11 in]
          n164 = call "BRig_dataLC_Selection_First_Block_l1.vi"() -> ("output_Selection_First_Block"=w540:i32)  [unwired: 11 in]
          n165 = call "BRig_dataLC_Selection_First_Count_l1.vi"() -> ("output_Selection_First_Count"=w541:i32)  [unwired: 11 in]
          n166 = call "BRig_dataLC_Selection_First_Prob_l1.vi"() -> ("output_Selection_First_Prob"=w542:i32)  [unwired: 11 in]
          n167 = call "BRig_dataLC_Selection_First_Delay_l1.vi"() -> ("output_Selection_First_Delay"=w543:i32)  [unwired: 11 in]
          n168 = call "BRig_dataLC_Selection_First_OnOff_l2.vi"() -> ("output_Selection_First_OnOff_l2"=w546:i32)  [unwired: 11 in]
          n169 = call "BRig_dataLC_Selection_First_Block_l2.vi"() -> ("output_Selection_First_Block_l2"=w544:i32)  [unwired: 11 in]
          n170 = call "BRig_dataLC_Selection_First_Count_l2.vi"() -> ("output_Selection_First_Count_l2"=w545:i32)  [unwired: 11 in]
          n171 = call "BRig_dataLC_Selection_First_Prob_l2.vi"() -> ("output_Selection_First_Prob_l2"=w538:i32)  [unwired: 11 in]
          n172 = call "BRig_dataLC_Selection_First_Delay_l2.vi"() -> ("output_Selection_First_Delay_l2"=w539:i32)  [unwired: 11 in]
        }
        frame 2 {
          n173 = call "BRig_dataLC_Selection_PreR_OnOff_l1.vi"() -> ("output_Selection_PreR_OnOff"=w557:i32)  [unwired: 11 in]
          n174 = call "BRig_dataLC_Selection_PreR_Block_l1.vi"() -> ("output_Selection_PreR_Block"=w555:i32)  [unwired: 11 in]
          n175 = call "BRig_dataLC_Selection_PreR_Count_l1.vi"() -> ("output_Selection_PreR_Count"=w554:i32)  [unwired: 11 in]
          n176 = call "BRig_dataLC_Selection_PreR_Prob_l1.vi"() -> ("output_Selection_PreR_Prob"=w553:i32)  [unwired: 11 in]
          n177 = call "BRig_dataLC_Selection_PreR_Delay_l1.vi"() -> ("output_Selection_PreR_Delay"=w552:i32)  [unwired: 11 in]
          n178 = call "BRig_dataLC_Selection_PreR_OnOff_l2.vi"() -> ("output_Selection_PreR_OnOff_l2"=w556:i32)  [unwired: 11 in]
          n179 = call "BRig_dataLC_Selection_PreR_Block_l2.vi"() -> ("output_Selection_PreR_Block_l2"=w551:i32)  [unwired: 11 in]
          n180 = call "BRig_dataLC_Selection_PreR_Count_l2.vi"() -> ("output_Selection_PreR_Count_l2"=w550:i32)  [unwired: 11 in]
          n181 = call "BRig_dataLC_Selection_PreR_Prob_l2.vi"() -> ("output_Selection_PreR_Prob_l2"=w549:i32)  [unwired: 11 in]
          n182 = call "BRig_dataLC_Selection_PreR_Delay_l2.vi"() -> ("output_Selection_PreR_Delay_l2"=w548:i32)  [unwired: 11 in]
        }
        frame 3 {
          n183 = call "BRig_dataLC_Selection_PostR_OnOff_l1.vi"() -> ("output_Selection_PostR_OnOff"=w567:i32)  [unwired: 11 in]
          n184 = call "BRig_dataLC_Selection_PostR_Block_l1.vi"() -> ("output_Selection_PostR_Block"=w558:i32)  [unwired: 11 in]
          n185 = call "BRig_dataLC_Selection_PostR_Count_l1.vi"() -> ("output_Selection_PostR_Count"=w565:i32)  [unwired: 11 in]
          n186 = call "BRig_dataLC_Selection_PostR_Prob_l1.vi"() -> ("output_Selection_PostR_Prob"=w564:i32)  [unwired: 11 in]
          n187 = call "BRig_dataLC_Selection_PostR_Delay_l1.vi"() -> ("output_Selection_PostR_Delay"=w563:i32)  [unwired: 11 in]
          n188 = call "BRig_dataLC_Selection_PostR_OnOff_l2.vi"() -> ("output_Selection_PostR_OnOff_l2"=w566:i32)  [unwired: 11 in]
          n189 = call "BRig_dataLC_Selection_PostR_Block_l2.vi"() -> ("output_Selection_PostR_Block_l2"=w562:i32)  [unwired: 11 in]
          n190 = call "BRig_dataLC_Selection_PostR_Count_l2.vi"() -> ("output_Selection_PostR_Count_l2"=w561:i32)  [unwired: 11 in]
          n191 = call "BRig_dataLC_Selection_PostR_Prob_l2.vi"() -> ("output_Selection_PostR_Prob_l2"=w560:i32)  [unwired: 11 in]
          n192 = call "BRig_dataLC_Selection_PostR_Delay_l2.vi"() -> ("output_Selection_PostR_Delay_l2"=w559:i32)  [unwired: 11 in]
        }
      }
      n193 = Less?(x=w251, y=u16 3) -> (x < y?=w298:bool)
      n194 = Select(t=w297, s=w298, f=w296) -> (s? t:f=w250:u16)
      n195 = Select(t=u16 0, s=w247, f=w250) -> (s? t:f=w249:u16)
      n196 = Boolean To (0,1)(Boolean=w292) -> (0, 1=w324:i16)
      n197 = Select(t=i16 2, s=w291, f=i16 0) -> (s? t:f=w325:i16)
      n198 = Add(x=w324, y=w325) -> (x+y=w289:i16)
      n199 = case shown="False" w247 {
        tunnel: w289 -> [w356 w457]
        tunnel: w288 -> [w355 w458]
        tunnel: w287 -> [w354 w455]
        tunnel: w286 -> [w353 w454]
        tunnel: w285 -> [w352 w453]
        tunnel: w284 -> [w351 w452]
        tunnel: w283 -> [w350 w451]
        tunnel: w282 -> [w349 w450]
        tunnel: w281 -> [w348 w449]
        tunnel: w280 -> [w347 w448]
        tunnel: w279 -> [w346 w447]
        tunnel: w278 -> [w345 w446]
        tunnel: w277 -> [w344 w445]
        tunnel: w276 -> [w343 w459]
        tunnel: w275 -> [w342 w460]
        tunnel: w274 -> [w341 w461]
        tunnel: [w340 w444] -> w273
        tunnel: [w339 w443] -> w272
        tunnel: [w338 w442] -> w271
        tunnel: [w337 w441] -> w270
        tunnel: [w336 w440] -> w269
        tunnel: [w335 w439] -> w268
        tunnel: [w334 w438] -> w267
        tunnel: [w333 w437] -> w266
        tunnel: w249 -> [w332 w456]
        frame False {
          n200 = case shown="3" w356 {
            tunnel: w355 -> [_ w379 w401 w436]
            tunnel: w343 -> [_ w372 w394 w424]
            tunnel: w354 -> [_ w373 w395 w425]
            tunnel: w332 -> [_ w371 w393 w423]
            tunnel: [w357 w370 w383 w422] -> w340
            tunnel: [w357 w369 w383 w421] -> w339
            tunnel: [w358 w368 w382 w420] -> w338
            tunnel: [w358 w367 w382 w419] -> w337
            tunnel: [w357 w361 w392 w418] -> w335
            tunnel: [w358 w359 w391 w417] -> w334
            tunnel: [w357 w361 w390 w416] -> w336
            tunnel: [w358 w359 w389 w415] -> w333
            tunnel: w353 -> [_ w366 _ w414]
            tunnel: w352 -> [_ w365 _ w413]
            tunnel: w351 -> [_ w364 _ w412]
            tunnel: w350 -> [_ w363 _ w411]
            tunnel: w349 -> [_ w362 _ w410]
            tunnel: w348 -> [_ _ w388 w409]
            tunnel: w347 -> [_ _ w387 w408]
            tunnel: w346 -> [_ _ w386 w407]
            tunnel: w345 -> [_ _ w385 w406]
            tunnel: w344 -> [_ _ w384 w405]
            tunnel: w341 -> [_ w360 _ w404]
            tunnel: w342 -> [_ _ w381 w403]
            frame 0, Default {
              w358 = u16 0
              w357 = FALSE
              # "No active lasers"
            }
            frame 1 {
              w359 = u16 0
              w361 = FALSE
              # "laser1 is active"
              n201 = Index Array(array=w379, index #1=w366, index #2=w365, index #3=w364, index #4=w363, index #5=w362) -> (element #1=w378:u16, element #2=w377:u16, element #3=w376:u16, element #4=w375:u16, element #5=w374:u16)
              n202 = call "BRig_RT__Case_Exp__State_initTrial__LC.vi"("input_L_OnOff"=w378, "input_L_Block"=w377, "input_L_Count"=w376, "input_L_Prob"=w375, "input_L_Tdelay"=w374, "input_L_delayOpt"=w359, "input_T_state"=w373, "input_iSpout"=w372, "input_iTrial_relative"=w371, "input_L_T"=w360) -> ("output_LC_Event"=w370:bool, "output_LC_Laser"=w369:bool, "output_L_Tstart"=w368:u16, "output_L_Tend"=w367:u16)  [unwired: 6 in]
            }
            frame 2 {
              w382 = u16 0
              w383 = FALSE
              # "laser2 is active"
              n203 = Index Array(array=w401, index #1=w388, index #2=w387, index #3=w386, index #4=w385, index #5=w384) -> (element #1=w396:u16, element #2=w397:u16, element #3=w398:u16, element #4=w399:u16, element #5=w400:u16)
              n204 = call "BRig_RT__Case_Exp__State_initTrial__LC.vi"("input_L_OnOff"=w396, "input_L_Block"=w397, "input_L_Count"=w398, "input_L_Prob"=w399, "input_L_Tdelay"=w400, "input_L_delayOpt"=u16 0, "input_T_state"=w395, "input_iSpout"=w394, "input_iTrial_relative"=w393, "input_L_T"=w381) -> ("output_LC_Event"=w390:bool, "output_LC_Laser"=w392:bool, "output_L_Tstart"=w391:u16, "output_L_Tend"=w389:u16)  [unwired: 6 in]
            }
            frame 3 {
              w402 = u16 0 ("input_L_delayOpt")
              # "laser1 and laser2 are active"
              n205 = Index Array(array=w436, index #1=w414, index #2=w413, index #3=w412, index #4=w411, index #5=w410, index #7=w409, index #8=w408, index #9=w407, index #10=w406, index #11=w405) -> (element #1=w435:u16, element #2=w434:u16, element #3=w433:u16, element #4=w432:u16, element #5=w431:u16, element #7=w426:u16, element #8=w427:u16, element #9=w428:u16, element #10=w429:u16, element #11=w430:u16)  [unwired: 1 in, 1 out]
              n206 = call "BRig_RT__Case_Exp__State_initTrial__LC.vi"("input_L_OnOff"=w435, "input_L_Block"=w434, "input_L_Count"=w433, "input_L_Prob"=w432, "input_L_Tdelay"=w431, "input_L_delayOpt"=w402, "input_T_state"=w425, "input_iSpout"=w424, "input_iTrial_relative"=w423, "input_L_T"=w404) -> ("output_LC_Event"=w422:bool, "output_LC_Laser"=w421:bool, "output_L_Tstart"=w420:u16, "output_L_Tend"=w419:u16)  [unwired: 6 in]
              n207 = call "BRig_RT__Case_Exp__State_initTrial__LC.vi"("input_L_OnOff"=w426, "input_L_Block"=w427, "input_L_Count"=w428, "input_L_Prob"=w429, "input_L_Tdelay"=w430, "input_L_delayOpt"=w402, "input_T_state"=w425, "input_iSpout"=w424, "input_iTrial_relative"=w423, "input_L_T"=w403) -> ("output_LC_Event"=w416:bool, "output_LC_Laser"=w418:bool, "output_L_Tstart"=w417:u16, "output_L_Tend"=w415:u16)  [unwired: 6 in]
            }
          }
        }
        frame True {
          n208 = case shown="3" w457 {
            tunnel: w458 -> [_ w483 w504 w537]
            tunnel: w459 -> [_ w464 w484 w505]
            tunnel: w455 -> [_ w478 w499 w528]
            tunnel: w456 -> [_ w477 w498 w527]
            tunnel: [w462 w476 w488 w526] -> w444
            tunnel: [w462 w475 w488 w525] -> w443
            tunnel: [w463 w474 w487 w524] -> w442
            tunnel: [w463 w473 w487 w523] -> w441
            tunnel: [w462 w467 w497 w522] -> w439
            tunnel: [w463 w465 w496 w521] -> w438
            tunnel: [w462 w467 w495 w520] -> w440
            tunnel: [w463 w465 w494 w519] -> w437
            tunnel: w454 -> [_ w472 _ w518]
            tunnel: w453 -> [_ w471 _ w517]
            tunnel: w452 -> [_ w470 _ w516]
            tunnel: w451 -> [_ w469 _ w515]
            tunnel: w450 -> [_ w468 _ w514]
            tunnel: w449 -> [_ _ w493 w513]
            tunnel: w448 -> [_ _ w492 w512]
            tunnel: w447 -> [_ _ w491 w511]
            tunnel: w446 -> [_ _ w490 w510]
            tunnel: w445 -> [_ _ w489 w509]
            tunnel: w461 -> [_ w466 _ w508]
            tunnel: w460 -> [_ _ w486 w507]
            frame 0, Default {
              w463 = u16 0
              w462 = FALSE
              # "No active lasers"
            }
            frame 1 {
              w465 = u16 0
              w467 = FALSE
              # "laser1 is active"
              n209 = Index Array(array=w483, index #1=w472, index #2=w471, index #3=w470, index #4=w469, index #5=w468) -> (element #1=w482:u16, element #3=w481:u16, element #4=w480:u16, element #5=w479:u16)  [unwired: 1 out]
              n210 = call "BRig_RT__Case_Exp__State_initTrial__LC.vi"("input_L_OnOff"=w482, "input_L_Block"=w464, "input_L_Count"=w481, "input_L_Prob"=w480, "input_L_Tdelay"=w479, "input_L_delayOpt"=w465, "input_T_state"=w478, "input_iSpout"=w464, "input_iTrial_relative"=w477, "input_L_T"=w466) -> ("output_LC_Event"=w476:bool, "output_LC_Laser"=w475:bool, "output_L_Tstart"=w474:u16, "output_L_Tend"=w473:u16)  [unwired: 6 in]
            }
            frame 2 {
              w487 = u16 0
              w488 = FALSE
              # "laser2 is active"
              n211 = Index Array(array=w504, index #1=w493, index #2=w492, index #3=w491, index #4=w490, index #5=w489) -> (element #1=w500:u16, element #3=w501:u16, element #4=w502:u16, element #5=w503:u16)  [unwired: 1 out]
              n212 = call "BRig_RT__Case_Exp__State_initTrial__LC.vi"("input_L_OnOff"=w500, "input_L_Block"=w484, "input_L_Count"=w501, "input_L_Prob"=w502, "input_L_Tdelay"=w503, "input_L_delayOpt"=u16 0, "input_T_state"=w499, "input_iSpout"=w484, "input_iTrial_relative"=w498, "input_L_T"=w486) -> ("output_LC_Event"=w495:bool, "output_LC_Laser"=w497:bool, "output_L_Tstart"=w496:u16, "output_L_Tend"=w494:u16)  [unwired: 6 in]
            }
            frame 3 {
              w506 = u16 0 ("input_L_delayOpt")
              # "laser1 and laser2 are active"
              n213 = Index Array(array=w537, index #1=w518, index #2=w517, index #3=w516, index #4=w515, index #5=w514, index #7=w513, index #8=w512, index #9=w511, index #10=w510, index #11=w509) -> (element #1=w536:u16, element #3=w535:u16, element #4=w534:u16, element #5=w533:u16, element #7=w529:u16, element #9=w530:u16, element #10=w531:u16, element #11=w532:u16)  [unwired: 1 in, 3 out]
              n214 = call "BRig_RT__Case_Exp__State_initTrial__LC.vi"("input_L_OnOff"=w536, "input_L_Block"=w505, "input_L_Count"=w535, "input_L_Prob"=w534, "input_L_Tdelay"=w533, "input_L_delayOpt"=w506, "input_T_state"=w528, "input_iSpout"=w505, "input_iTrial_relative"=w527, "input_L_T"=w508) -> ("output_LC_Event"=w526:bool, "output_LC_Laser"=w525:bool, "output_L_Tstart"=w524:u16, "output_L_Tend"=w523:u16)  [unwired: 6 in]
              n215 = call "BRig_RT__Case_Exp__State_initTrial__LC.vi"("input_L_OnOff"=w529, "input_L_Block"=w505, "input_L_Count"=w530, "input_L_Prob"=w531, "input_L_Tdelay"=w532, "input_L_delayOpt"=w506, "input_T_state"=w528, "input_iSpout"=w505, "input_iTrial_relative"=w527, "input_L_T"=w507) -> ("output_LC_Event"=w520:bool, "output_LC_Laser"=w522:bool, "output_L_Tstart"=w521:u16, "output_L_Tend"=w519:u16)  [unwired: 6 in]
            }
          }
        }
      }
      n216 = call "BRig_dataCurrent_L_Sel_T_start_l1.vi"() -> ("output_L_Sel_T_start_l1"=w265:i32)  [unwired: 11 in]
      n217 = call "BRig_dataCurrent_L_Sel_T_end_l1.vi"() -> ("output_L_Sel_T_end_l1"=w264:i32)  [unwired: 11 in]
      n218 = call "BRig_dataCurrent_L_Sel_T_start_l2.vi"() -> ("output_L_Sel_T_start_l2"=w263:i32)  [unwired: 11 in]
      n219 = call "BRig_dataCurrent_L_Sel_T_end_l2.vi"() -> ("output_L_Sel_T_end_l2"=w262:i32)  [unwired: 11 in]
      n220 = Replace Array Subset(array=w310, new element #1=w271, index #1=w265, new element #2=w270, index #2=w264, new element #3=w267, index #3=w263, new element #4=w266, index #4=w262) -> (w309:u16[])
      n221 = call "BRig_dataTrial_L_Sel_event_I_l1.vi"() -> ("output_L_Sel_event_I_l1"=w257:i32)  [unwired: 11 in]
      n222 = call "BRig_dataTrial_L_Sel_trig_I_l1.vi"() -> ("output_L_Sel_trig_I_l1"=w256:i32)  [unwired: 11 in]
      n223 = call "BRig_dataTrial_L_Sel_event_I_l2.vi"() -> ("output_L_Sel_event_I_l2"=w255:i32)  [unwired: 11 in]
      n224 = call "BRig_dataTrial_L_Sel_trig_I_l2.vi"() -> ("output_L_Sel_trig_I_l2"=w254:i32)  [unwired: 11 in]
      n225 = call "BRig_arrTrig_L_Selection_event_l1.vi"() -> ("output_L_Sel_event_l1"=w261:i32)  [unwired: 11 in]
      n226 = call "BRig_arrTrig_L_Selection_laser_l1.vi"() -> ("output_L_Sel_laserTrig_l1"=w260:i32)  [unwired: 11 in]
      n227 = call "BRig_arrTrig_L_Selection_event_l2.vi"() -> ("output_L_Sel_event_l2"=w259:i32)  [unwired: 11 in]
      n228 = call "BRig_arrTrig_L_Selection_laser_l2.vi"() -> ("output_L_Sel_laserTrig_l2"=w258:i32)  [unwired: 11 in]
      n229 = Boolean To (0,1)(Boolean=w273) -> (0, 1=w319:i16)
      n230 = Boolean To (0,1)(Boolean=w272) -> (0, 1=w318:i16)
      n231 = Boolean To (0,1)(Boolean=w269) -> (0, 1=w316:i16)
      n232 = Boolean To (0,1)(Boolean=w268) -> (0, 1=w317:i16)
      n233 = Replace Array Subset(array=w321, new element #1=w273, index #1=w261, new element #2=w272, index #2=w260, new element #3=w269, index #3=w259, new element #4=w268, index #4=w258) -> (w320:bool[])
      n234 = To Unsigned Word Integer(number=w319) -> (unsigned 16bit integer=w315:u16)
      n235 = To Unsigned Word Integer(number=w318) -> (unsigned 16bit integer=w314:u16)
      n236 = To Unsigned Word Integer(number=w316) -> (unsigned 16bit integer=w313:u16)
      n237 = To Unsigned Word Integer(number=w317) -> (unsigned 16bit integer=w312:u16)
      n238 = Replace Array Subset(array=w300, new element #1=w315, index (row) #1=w303, index (col) #1=w257, new element #2=w314, index (row) #2=w303, index (col) #2=w256, new element #3=w313, index (row) #3=w303, index (col) #3=w255, new element #4=w312, index (row) #4=w303, index (col) #4=w254) -> (w311:u16[][])
    }
  }
  "output_dataCurrent" <- w10
  "output_arrTrig" <- w13
  "output_dataTrial" <- w12
